vi "ObtainTCPSocket.vi"(7 "write (f)":bool, 8 "ErrorArray":errorcluster[](array[cluster]), 10 "timeout":i32=10000, 11 "SocketRef":refnum<class "Socket.TCP.lvclass">) -> (0 "ErrorArray":errorcluster[](array[cluster]), 3 "SocketRef":refnum<class "Socket.TCP.lvclass">)   [LabVIEW 2017, in "Comms.lvlib"]
uses:
  Comms.lvlib
  <userlib>/NIST/Socket Class/Classes/Socket.TCP/Socket.TCP.lvclass
  C:/Program Files (x86)/National Instruments/LabVIEW 2017/user.lib/NIST/Socket Class/Classes/Socket.Base/Socket.Base.lvclass
  <userlib>/NIST/Socket Class/Classes/Socket.Base/Socket.Base.lvclass/Socket.Base.ctl
  <userlib>/NIST/Socket Class/Classes/Socket.Base/Accessors/Read initialized.vi
  <userlib>/NIST/NISTErrorLib/NISTErrorLib.lvlib
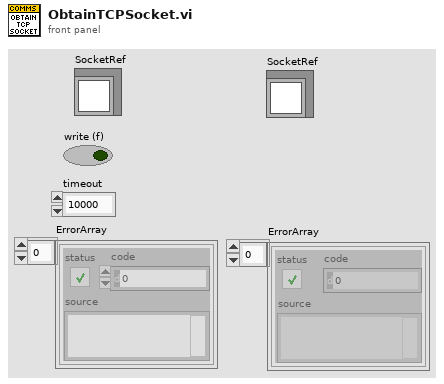
[diagram p1: front panel]
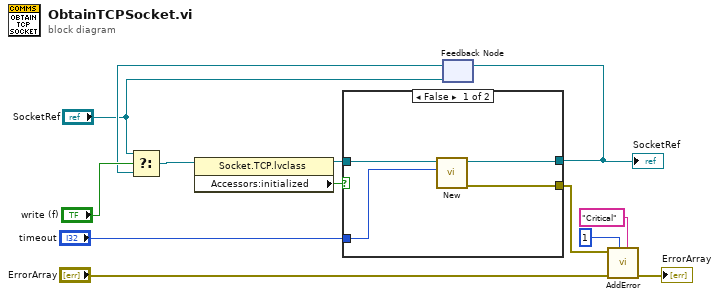
[diagram p0: block diagram]
diagram:
  n1 = feedback #1("SocketRef") -> (w2:refnum<class "Socket.TCP.lvclass">)
  n2 = Select(t="SocketRef", s="write (f)", f=w2) -> (s? t:f=w3:refnum<class "Socket.TCP.lvclass">)
  n3 = property class="Socket.TCP.lvclass"(reference=w3) -> (reference out=w10:refnum<class "Socket.TCP.lvclass">, "Accessors:initialized"=w9:bool)  [unwired: 1 in, 1 out]
  n4 = case shown="False" w9 {
    tunnel: [w17 w18] -> w11
    tunnel: w10 -> [w16 w18]
    tunnel: "timeout" -> [w15 _]
    tunnel: [w14 _] -> w7
    frame False {
      n5 = call-dynamic "New.vi"("timeout"=w15, "Socket.TCP in"=w16) -> ("error out"=w14:errorcluster, "Socket.TCP out"=w17:refnum<class "Socket.TCP.lvclass">)  [unwired: 8 in]
    }
    frame True {
    }
  }
  "SocketRef" <- w11
  n6 = feedback-in #1(w11) -> ()
  n7 = call <userlib>:"AddError.vi"("Severity"="Critical", "Priority"=u8 1, "ErrorArray"="ErrorArray", "error in (no error)"=w7) -> ("ErrorArray"=→"ErrorArray":errorcluster[])  [unwired: 6 in, 1 out]
